vi "createMotionProfile.vi"(6 "ms per frame":dbl=50.0, 8 "Max Jerk (In/sec^3)":dbl=60.0, 9 "Max Acceleration (In/sec^2)":dbl=80.0, 10 "Max Speed (In/sec)":dbl=120.0, 11 "Inches to Travel":dbl=250.0) -> (3 "Profile":T1)   [LabVIEW 2015]
panel:
  out "Final Position":dbl
  out "XY Graph":cluster{dbl[], dbl[]}[](graph)
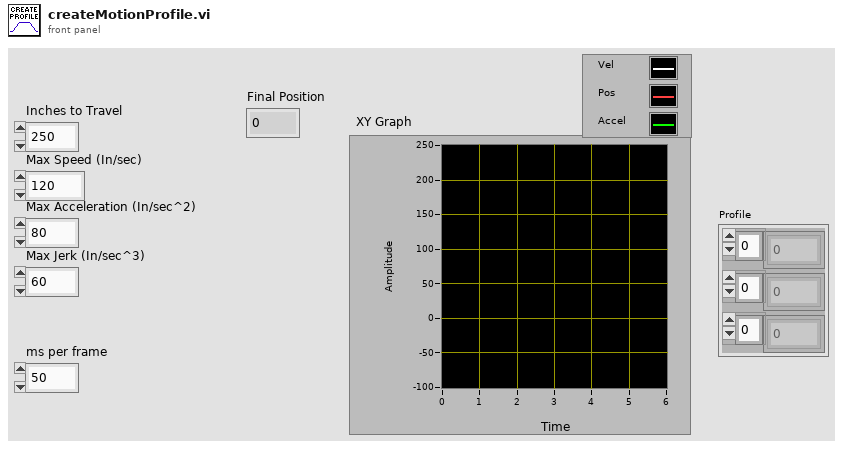
[diagram p1: front panel]
types:
  T1 = cluster{"Positions":dbl[], "Velocities":dbl[], "Accelerations":dbl[]}
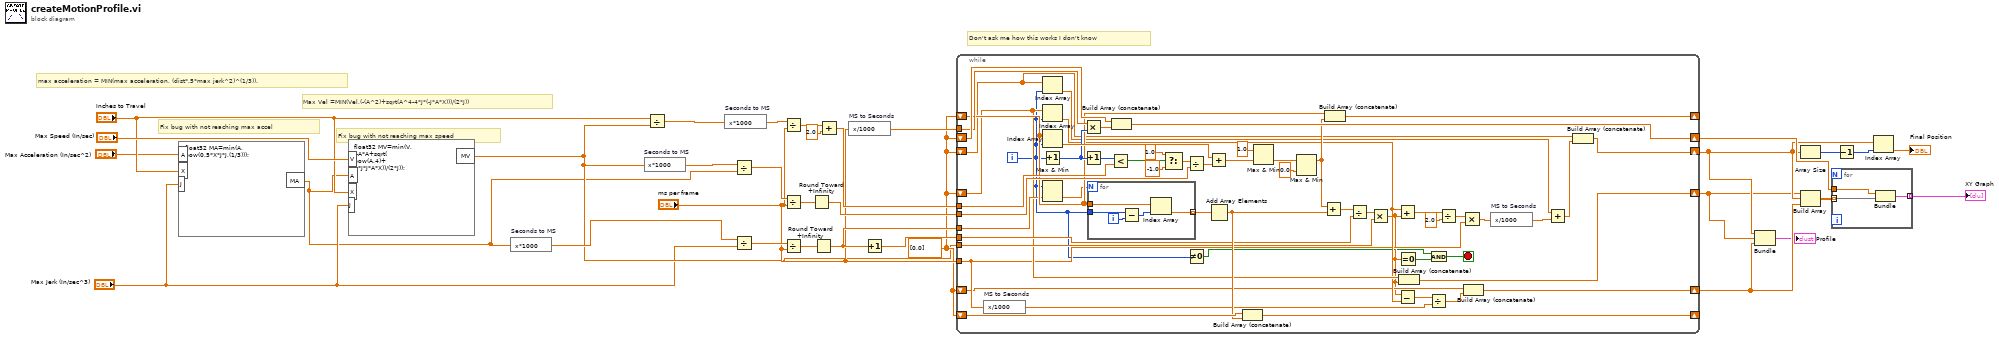
[diagram p0: block diagram]
diagram:
  w17 = dbl[] [0.0]
  # "Fix bug with not reaching max accel"
  # "max acceleration = MIN(max acceleration, (dist*.5*max jerk^2)^(1/3))."
  # "Don't ask me how this works I don't know"
  # "Fix bug with not reaching max speed"
  # "Max Vel =MIN(Vel,(-(A^2)+sqrt(A^4-4*J*(-J*A*X)))/(2*J))"
  n1 = formula code="float32 MA=min(A,\npow(0.5*X*J*J,(1/3)));"("A"="Max Acceleration (In/sec^2)", "X"="Inches to Travel", "J"="Max Jerk (In/sec^3)") -> ("MA"=w5:sgl)
  n2 = formula code="float32 MV=min(V,\n(-A*A+sqrt(\npow(A,4)+\n4*J*J*A*X))/(2*J));"("V"="Max Speed (In/sec)", "A"=w5, "X"="Inches to Travel", "J"="Max Jerk (In/sec^3)") -> ("MV"=w10:sgl)
  n3 = expression code="x*1000" "Seconds to MS"(w5) -> (w32:sgl)
  n4 = expression code="x*1000" "Seconds to MS"(w10) -> (w31:sgl)
  n5 = Divide(x="Inches to Travel", y=w10) -> (x/y=w30:dbl)
  n6 = expression code="x*1000" "Seconds to MS"(w30) -> (w29:dbl)
  n7 = Divide(x=w31, y=w5) -> (x/y=w25:sgl)
  n8 = Divide(x=w32, y="Max Jerk (In/sec^3)") -> (x/y=w22:dbl)
  n9 = Divide(x=w29, y="ms per frame") -> (x/y=w28:dbl)
  n10 = Divide(x=w25, y="ms per frame") -> (x/y=w24:dbl)
  n11 = Divide(x=w22, y="ms per frame") -> (x/y=w21:dbl)
  n12 = Round Toward +Infinity(x=w24) -> (ceil(x): smallest int >= x=w23:dbl)
  n13 = Round Toward +Infinity(x=w21) -> (ceil(x): smallest int >= x=w20:dbl)
  n14 = Add(x=w28, y=2.0) -> (x+y=w26:dbl)
  n15 = expression code="x/1000" "MS to Seconds"("ms per frame") -> (w33:dbl)
  n16 = Increment(x=w20) -> (x+1=w19:dbl)
  n17 = while {
    shift-right: [w86] -> w15
    shift-left: w17 -> [w87]
    tunnel: w33 -> [w85]
    tunnel: w26 -> [w83]
    shift-right: [w69] -> _
    shift-left: w17 -> [w68]
    tunnel: w23 -> [w75]
    tunnel: w20 -> [w66]
    shift-right: [w63] -> _
    shift-left: w17 -> [w64]
    tunnel: w19 -> [w59]
    tunnel: w10 -> [w57]
    shift-right: [w56] -> w1
    shift-left: w17 -> [w54]
    shift-right: [w55] -> w4
    shift-left: w17 -> [w48]
    tunnel: "ms per frame" -> [w42]
    shift-right: [w40] -> w3
    shift-left: w17 -> [w39]
    i -> [w38]
    stop <- w34 stop-if-true
    n18 = expression code="x/1000" "MS to Seconds"(w42) -> (w43:dbl)
    n19 = Index Array(array=w48, index=w38) -> (element=w47:dbl)
    n20 = Index Array(array=w54, index=w38) -> (element=w45:dbl)
    n21 = Index Array(array=w68, index=w38) -> (element=w73:dbl)
    n22 = Increment(x=w38) -> (x+1=w71:i32)
    n23 = Max & Min(x=w38, y=w66) -> (min(x,y)=w65:dbl)  [unwired: 1 out]
    n24 = Multiply(x=w85, y=w71) -> (x*y=w84:dbl)
    n25 = Increment(x=w71) -> (x+1=w72:i32)
    n26 = for {
      N: w65 -> [_]
      tunnel: w38 -> [w91]
      tunnel: w68 -> [w89]
      tunnel: [w88] -> w67 mode=indexing
      i -> [w92]
      n27 = Subtract(x=w91, y=w92) -> (x-y=w90:i32)
      n28 = Index Array(array=w89, index=w90) -> (element=w88:dbl)
    }
    n29 = Less?(x=w72, y=w83) -> (x < y?=w79:bool)
    n30 = Build Array (concatenate)(w87, w84) -> (w86:dbl[])
    n31 = Select(t=1.0, s=w79, f=-1.0) -> (s? t:f=w76:dbl)
    n32 = Divide(x=w76, y=w75) -> (x/y=w74:dbl)
    n33 = Not Equal To 0?(x=w38) -> (x != 0?=w35:bool)
    n34 = Add(x=w73, y=w74) -> (x+y=w70:dbl)
    n35 = Add Array Elements(numeric array=w67) -> (sum=w62:dbl)
    n36 = Build Array (concatenate)(w64, w62) -> (w63:dbl[])
    n37 = Max & Min(x=1.0, y=w70) -> (min(x,y)=w81:dbl)  [unwired: 1 out]
    n38 = Max & Min(x=w81, y=0.0) -> (max(x,y)=w61:dbl)  [unwired: 1 out]
    n39 = Add(x=w61, y=w62) -> (x+y=w60:dbl)
    n40 = Build Array (concatenate)(w68, w61) -> (w69:dbl[])
    n41 = Divide(x=w60, y=w59) -> (x/y=w58:dbl)
    n42 = Multiply(x=w58, y=w57) -> (x*y=w37:dbl)
    n43 = Add(x=w45, y=w37) -> (x+y=w53:dbl)
    n44 = Subtract(x=w37, y=w45) -> (x-y=w44:dbl)
    n45 = Equal To 0?(x=w37) -> (x = 0?=w36:bool)
    n46 = Build Array (concatenate)(w54, w37) -> (w56:dbl[])
    n47 = Divide(x=w44, y=w43) -> (x/y=w41:dbl)
    n48 = And(x=w35, y=w36) -> (x .and. y?=w34:bool)
    n49 = Divide(x=w53, y=2.0) -> (x/y=w51:dbl)
    n50 = Multiply(x=w51, y=w42) -> (x*y=w50:dbl)
    n51 = Build Array (concatenate)(w39, w41) -> (w40:dbl[])
    n52 = expression code="x/1000" "MS to Seconds"(w50) -> (w49:dbl)
    n53 = Add(x=w47, y=w49) -> (x+y=w46:dbl)
    n54 = Build Array (concatenate)(w48, w46) -> (w55:dbl[])
  }
  n55 = Bundle(w4, w1, w3) -> (→"Profile":cluster{dbl[], dbl[], dbl[]})  [unwired: 1 in]
  n56 = Array Size(array=w4) -> (size(s)=w13:i32)
  n57 = Build Array(w1, w4, w3) -> (w16:dbl[][])
  n58 = for {
    tunnel: w16 -> [w95] mode=indexing
    tunnel: w15 -> [w94]
    tunnel: [w93] -> w14 mode=indexing
    n59 = Bundle(w94, w95) -> (w93:cluster{dbl[], dbl[]})  [unwired: 1 in]
  }
  "XY Graph" <- w14
  n60 = Decrement(x=w13) -> (x-1=w12:i32)
  n61 = Index Array(array=w4, index=w12) -> (element=→"Final Position":dbl)
